vi "CSM - Module VI Ref.vi"(6 "Response Timeout(5000ms)":i32=5000, 7 "Target Module":string="A", 8 "Error In (no error)":errorcluster) -> (0 "error out":errorcluster, 3 "CSM VI Ref":refnum<vi>)   [LabVIEW 2017, in "API String Arguments Support.lvlib"]
doc: "This VI is oblselete. Please use \"CSM - Module VI Reference.vi\" instead."
uses:
  API String Arguments Support.lvlib
  <userlib>/_NEVSTOP/Communicable State Machine(CSM)/Communicable State Machine.lvlib
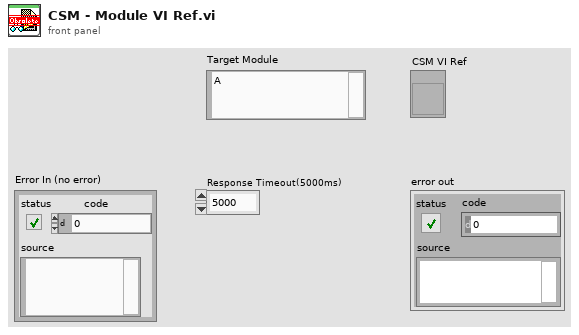
[diagram p1: front panel]
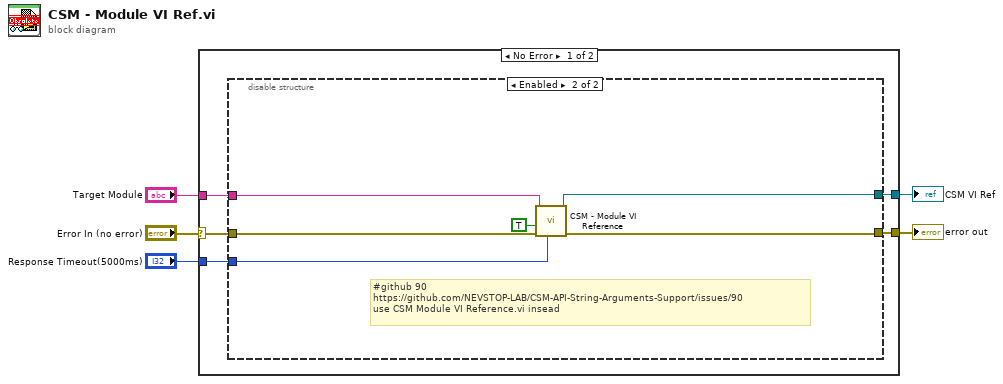
[diagram p0: block diagram]
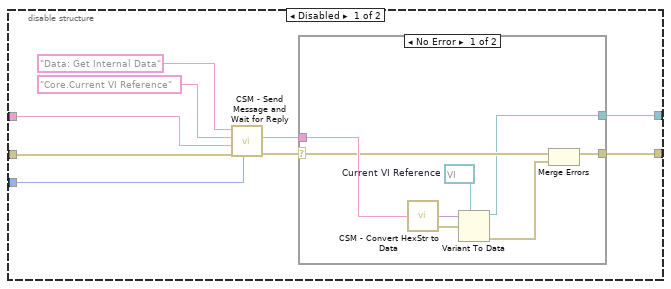
[diagram p2: hidden frame]
diagram:
  n1 = case shown="No Error" "Error In (no error)" {
    selector: "Error In (no error)" -> [w8 w35]
    tunnel: "Response Timeout(5000ms)" -> [w10 _]
    tunnel: [w9 w35] -> w4
    tunnel: [w7 _] -> w2
    tunnel: "Target Module" -> [w6 _]
    frame No Error {
      n2 = disable-structure shown="Enabled" {
        disable-tunnel: w10 -> [w18 w34]
        disable-tunnel: [w15 w31] -> w9
        disable-tunnel: w8 -> [w14 w33]
        disable-tunnel: [w12 w30] -> w7
        disable-tunnel: w6 -> [w11 w32]
        frame Disabled {
          n3 = call <userlib>:"CSM - Send Message and Wait for Reply.vi"("Response Timeout(-2 using Global Settings)"=w18, "Error In (no error)"=w14, "Target Module"=w11, "Arguments (\"\")"="Core.Current VI Reference" ("Name(\"\" to use uuid)"), "State"="Data: Get Internal Data") -> ("error out"=w16:errorcluster, "Response"=w17:string)  [unwired: 4 in, 1 out]
          n4 = case shown="No Error" w16 {
            selector: w16 -> [w22 w28]
            tunnel: w17 -> [w27 _]
            tunnel: [w23 w28] -> w15
            tunnel: [w20 _] -> w12
            frame No Error {
              w24 = refnum<vi> refnum  # Current VI Reference
              n5 = call <userlib>:"CSM - Convert HexStr to Data.vi"("HEX String"=w27) -> ("Variant"=w25:variant, "error out"=w26:errorcluster)  [unwired: 7 in]
              n6 = Variant To Data(error in=w26, type=w24, Variant=w25) -> (data=w20:refnum<vi>, error out=w21:errorcluster)
              n7 = Merge Errors(w22, w21) -> (w23:errorcluster)
            }
            frame Error {
            }
          }
        }
        frame Enabled {
          # "#github 90\nhttps://github.com/NEVSTOP-LAB/CSM-API-String-Arguments-Support/issues/90\nuse CSM Module VI Reference.vi insead"
          n8 = call <userlib>:"CSM - Module VI Reference.vi"("Response Timeout(-2 using Global Settings)"=w34, "error in (no error)"=w33, "force?(F)"=TRUE, "CSM Name"=w32) -> ("error out"=w31:errorcluster, "CSM Module VIRef"=w30:refnum<vi>)  [unwired: 6 in]
        }
      }
    }
    frame Error {
    }
  }
  "error out" <- w4
  "CSM VI Ref" <- w2
